vi "GetClassName.vi"(0 "reference in":refnum<class "G#Object.lvclass">, 5 "error in (no error)":errorcluster) -> (14 "reference out":refnum<class "G#Object.lvclass">, 15 "class name":string, 16 "lvlib hierarchy":string[](array[string]), 17 "full class name":string, 19 "error out":errorcluster)   [LabVIEW 2020, in "G#Object.lvclass"]
doc: "Returns the class name, full class name , lvlib hierarchy for the specified object."
uses:
  G#Object.lvclass
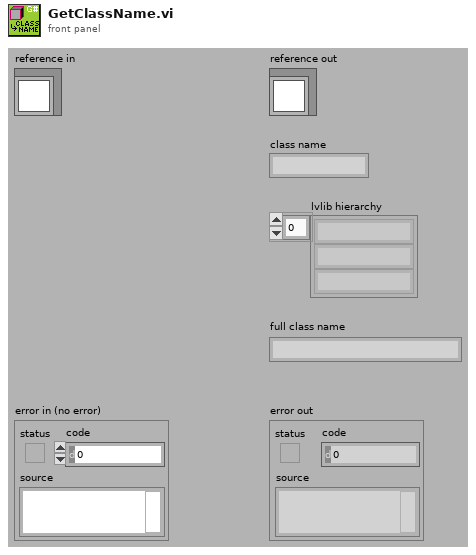
[diagram p1: front panel]
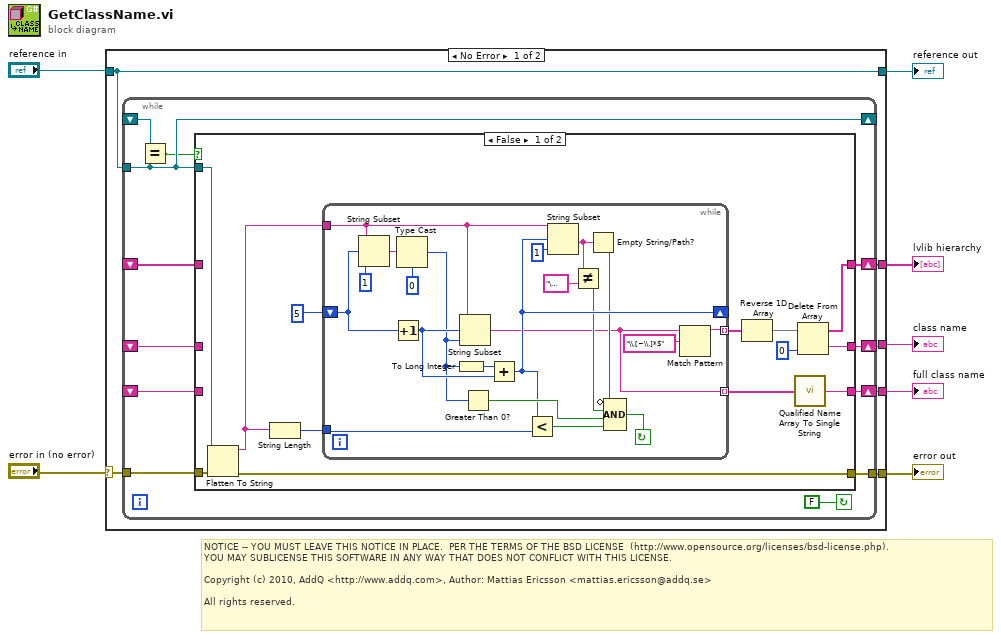
[diagram p0: block diagram]
diagram:
  # "NOTICE -- YOU MUST LEAVE THIS NOTICE IN PLACE.  PER THE TERMS OF THE BSD LICENSE  (http://www.opensource.org/licenses/bsd-license.php).\nYOU MAY SUBLICENSE THIS SOFTWARE IN ANY WAY THAT DOES NOT CONFLICT WITH THIS LICENSE.\n\nCopyright (c) 2010, AddQ <http://www.addq.com>, Author: Mattias Ericsson <mattias.ericsson@addq.se>\n\nAll rights reserved."
  n1 = case shown="No Error" "error in (no error)" {
    selector: "error in (no error)" -> [w12 w65]
    tunnel: "reference in" -> [w8 w64]
    tunnel: [w13 w65] -> w2
    tunnel: [w9 _] -> w6
    tunnel: [w10 _] -> w5
    tunnel: [w11 _] -> w4
    tunnel: [w8 w64] -> w1
    frame No Error {
      n2 = while {
        tunnel: [w25] -> w13
        tunnel: w12 -> [w24]
        tunnel: w8 -> [w18]
        shift-right: [w18] -> _
        shift-left: _ -> [w19]
        shift-right: [w21] -> w9
        shift-left: _ -> [w17]
        shift-right: [w22] -> w10
        shift-left: _ -> [w16]
        shift-right: [w23] -> w11
        shift-left: _ -> [w15]
        stop <- FALSE continue-if-true
        n3 = Equal?(x=w19, y=w18) -> (x = y?=w14:bool)
        n4 = case shown="False" w14 {
          tunnel: [w38 w61] -> w25
          tunnel: w24 -> [w37 w61]
          tunnel: [w33 w60] -> w23
          tunnel: [w30 w62] -> w22
          tunnel: [w29 w63] -> w21
          tunnel: w18 -> [w26 _]
          tunnel: w17 -> [_ w63]
          tunnel: w16 -> [_ w62]
          tunnel: w15 -> [_ w60]
          frame False {
            n5 = Flatten To String(anything=w26, error in (no error)=w37) -> (data string=w35:string, error out=w38:errorcluster)  [unwired: 2 in, 1 out]
            n6 = String Length(string=w35) -> (length=w34:i32)
            n7 = while {
              tunnel: w35 -> [w44]
              shift-right: [w48] -> _
              shift-left: 5 -> [w53]
              tunnel: w34 -> [w55]
              tunnel: [w40] -> w28 mode=indexing
              tunnel: [w39] -> w27 mode=indexing
              stop <- w54 continue-if-true
              n8 = String Subset(string=w44, offset (0)=w53, length (rest)=1 ("length (rest)")) -> (substring=w51:string)
              n9 = Increment(x=w53) -> (x+1=w59:i32)
              n10 = Type Cast(type=u8 0 ("default (0 U32)"), x=w51) -> (*(type *) &x=w49:u8)
              n11 = To Long Integer(number=w49) -> (32bit integer=w58:i32)
              n12 = String Subset(string=w44, offset (0)=w59, length (rest)=w49) -> (substring=w39:string)
              n13 = Greater Than 0?(x=w49) -> (x > 0?=w57:bool)
              n14 = Add(x=w58, y=w59) -> (x+y=w48:i32)
              n15 = Less?(x=w48, y=w55) -> (x < y?=w56:bool)
              n16 = String Subset(string=w44, offset (0)=w48, length (rest)=1 ("length (rest)")) -> (substring=w43:string)
              n17 = Not Equal?(x=w43, y="\u0000") -> (x != y?=w45:bool)
              n18 = Empty String/Path?(string/path=w43) -> (empty?=w42:bool)
              n19 = Compound Arithmetic op=AND(invert w42, w45, w57, w56) -> (w54:bool)
              n20 = Match Pattern(string=w39, regular expression="\\.[~\\.]*$") -> (before substring=w40:string)  [unwired: 4 out]
            }
            n21 = Reverse 1D Array(array=w28) -> (reversed array=w31:string[])
            n22 = call <vilib>:"Qualified Name Array To Single String.vi"("Fully Qualified Array"=w27) -> ("Fully Qualified String"=w33:string)
            n23 = Delete From Array(array=w31, index=0) -> (deleted portion=w30:string, array with subset deleted=w29:string[])  [unwired: 1 in]
          }
          frame True {
          }
        }
      }
    }
    frame Error {
    }
  }
  "reference out" <- w1
  "class name" <- w5
  "lvlib hierarchy" <- w6
  "full class name" <- w4
  "error out" <- w2
